vi "test-Vision-Utils-Test2.vi"() -> (3 "All Passed":bool)   [LabVIEW 2019]
uses:
  <vilib>/Rock Robotics/WPI/ThirdParty/JAS_Junk/TrajLib/Rotation_CreateAngle.vi
  <vilib>/Rock Robotics/WPI/ThirdParty/JAS_Junk/TrajLib/Rotation_GetAngleCosSin.vi
  <vilib>/Rock Robotics/WPI/ThirdParty/JAS_Junk/TrajLib/Rotation_UnaryMinus.vi
  <vilib>/Rock Robotics/WPI/ThirdParty/JAS_Junk/TrajLib/Rotation_Minus.vi
  <vilib>/Rock Robotics/WPI/ThirdParty/JAS_Junk/TrajLib/Pose_getRotation.vi
  <vilib>/Rock Robotics/WPI/ThirdParty/JAS_Junk/TrajLib/CompVisionUtil_EstimateFieldToCamera.vi
  <vilib>/Rock Robotics/WPI/ThirdParty/JAS_Junk/TrajLib/Pose_TransformBy.vi
  <vilib>/Rock Robotics/WPI/ThirdParty/JAS_Junk/TrajLib/Rotation_RotateBy.vi
  <vilib>/Rock Robotics/WPI/ThirdParty/JAS_Junk/TrajLib/Transform_Inverse.vi
  <vilib>/Rock Robotics/WPI/ThirdParty/JAS_Junk/TrajLib/Translation_RotateBy.vi
  <vilib>/Rock Robotics/WPI/ThirdParty/JAS_Junk/TrajLib/Translation_Plus.vi
  <vilib>/Rock Robotics/WPI/ThirdParty/JAS_Junk/TrajLib/Rotation_Plus.vi
  <vilib>/Rock Robotics/WPI/ThirdParty/JAS_Junk/TrajLib/Pose_New_TRRO.vi
  <vilib>/Rock Robotics/WPI/ThirdParty/JAS_Junk/TrajLib/Rotation_CreateXY.vi
  <vilib>/Rock Robotics/WPI/ThirdParty/JAS_Junk/TrajLib/Translation_UnaryMinus.vi
  <vilib>/Rock Robotics/WPI/ThirdParty/JAS_Junk/TrajLib/Util_CalcDist.vi
  <vilib>/Rock Robotics/WPI/ThirdParty/JAS_Junk/TrajLib/Trajectory_Library.lvlib
panel:
  out "Test 3":bool
  out "Test 2":bool
  out "Test 1":bool
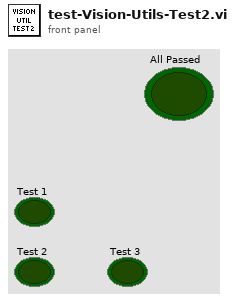
[diagram p1: front panel]
types:
  T1 = typedef "Trajectory_Library.lvlib/ROTATION2D.ctl" = cluster{"VALUE":dbl, "COS":dbl, "SIN":dbl}
  T2 = typedef "Trajectory_Library.lvlib/POSE2D.ctl" = cluster{"TRANSLATION":T3, "ROTATION":T1}
  T3 = typedef "Trajectory_Library.lvlib/TRANSLATION2D.ctl" = cluster{"X":dbl, "Y":dbl}
  T4 = typedef "Trajectory_Library.lvlib/TRANSFORM2D.ctl" = cluster{"TRANSLATION":T3, "ROTATION":T1}
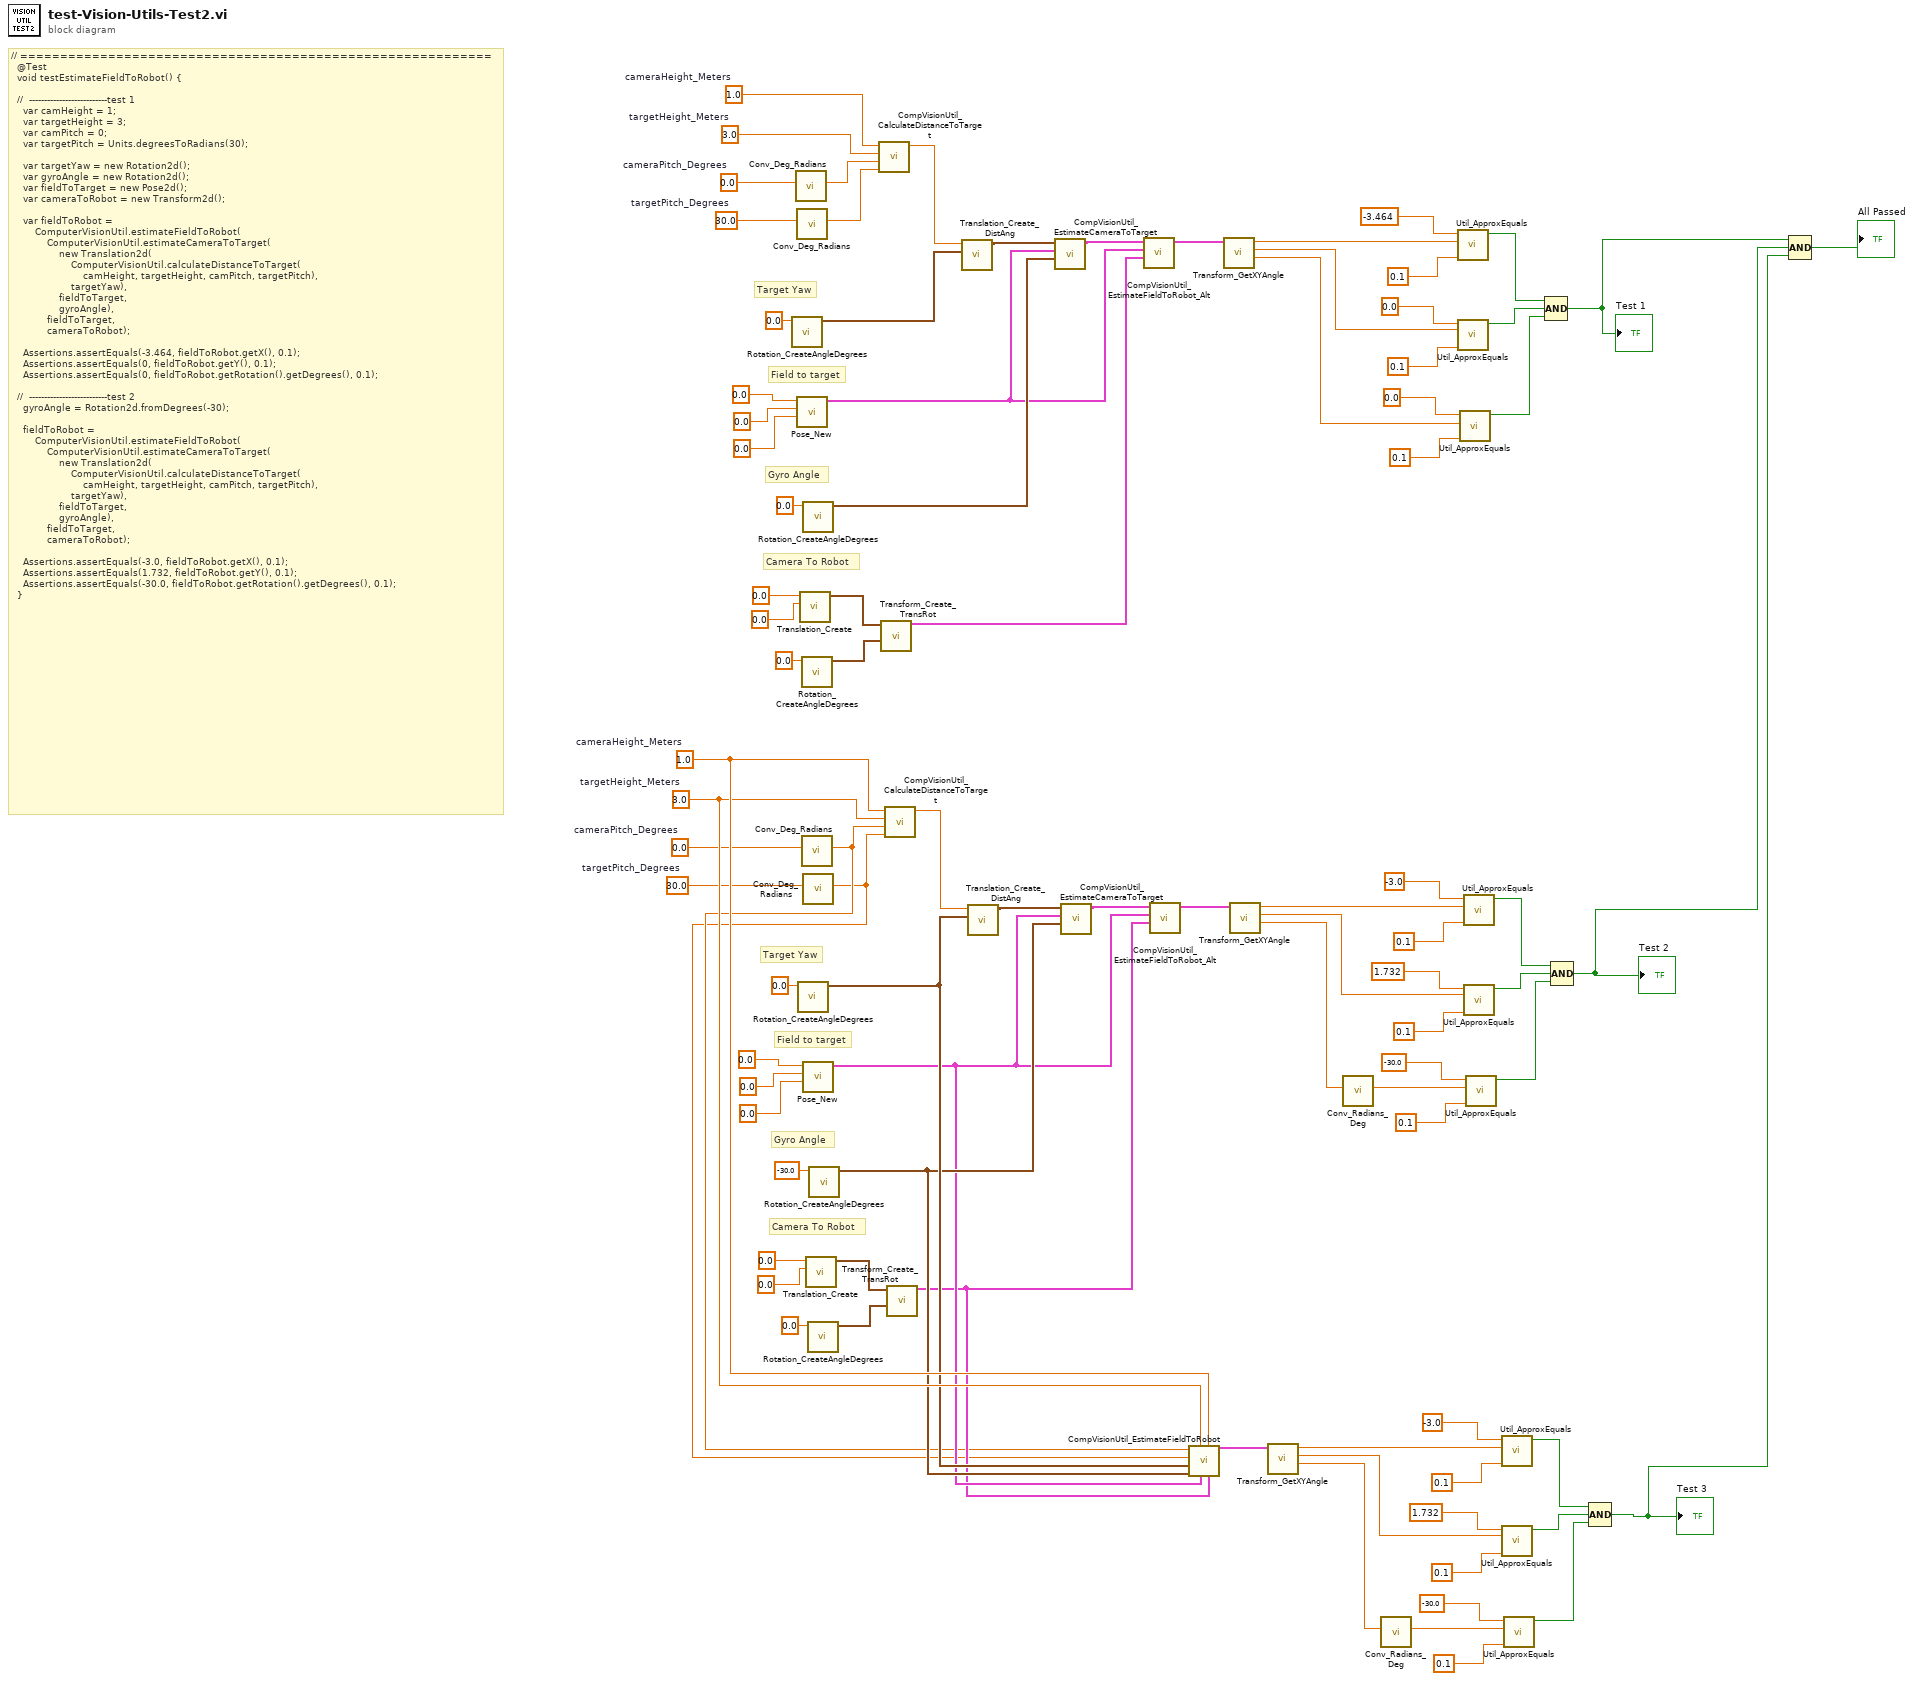
[diagram p0: block diagram]
diagram:
  w11 = 1.0  # cameraHeight_Meters
  w10 = 3.0  # targetHeight_Meters
  w9 = 0.0  # cameraPitch_Degrees
  w8 = 30.0  # targetPitch_Degrees
  w87 = 1.0  # cameraHeight_Meters
  w88 = 3.0  # targetHeight_Meters
  w86 = 0.0  # cameraPitch_Degrees
  w85 = 30.0  # targetPitch_Degrees
  # "Camera To Robot"
  # "Field to target"
  # "Gyro Angle"
  # "Target Yaw"
  # "Camera To Robot"
  # "Field to target"
  # "Gyro Angle"
  # "Target Yaw"
  # "// ===========================================================\n  @Test\n  void testEstimateFieldToRobot() {\n\n  //  --------------------------test 1\n    var camHeight = 1;\n    var targetHeight = 3;\n    var camPitch = 0;\n    var targetPitch = Units.degreesToRadians(30);\n\n    var targetYaw = new Rotation2d();\n    var gyroAngle = new Rotation2d();\n    var fieldToTarget = new Pose2d();\n    var cameraToRobot = new Transform2d();\n\n    var fieldToRobot =\n        ComputerVisionUtil.estimateFieldToRobot(\n            ComputerVisionUtil.estimateCameraToTarget(\n                new Translation2d(\n                    ComputerVisionUtil.calculateDistanceToTarget(\n                        camHeight, targetHeight, camPitch, targetPitch),\n                    targetYaw),\n                fieldToTarget,\n                gyroAngle),\n            fieldToTarget,\n            cameraToRobot);\n\n    Assertions.assertEquals(-3.464, fieldToRobot.getX(), 0.1);\n    Assertions.assertEquals(0, fieldToRobot.getY(), 0.1);\n    Assertions.assertEquals(0, fieldToRobot.getRotation().getDegrees(), 0.1);\n\n  //  --------------------------test 2\n    gyroAngle = Rotation2d.fromDegrees(-30);\n\n    fieldToRobot =\n        ComputerVisionUtil.estimateFieldToRobot(\n            ComputerVisionUtil.estimateCameraToTarget(\n                new Translation2d(\n                    ComputerVisionUtil.calculateDistanceToTarget(\n                        camHeight, targetHeight, camPitch, targetPitch),\n                    targetYaw),\n                fieldToTarget,\n                gyroAngle),\n            fieldToTarget,\n            cameraToRobot);\n\n    Assertions.assertEquals(-3.0, fieldToRobot.getX(), 0.1);\n    Assertions.assertEquals(1.732, fieldToRobot.getY(), 0.1);\n    Assertions.assertEquals(-30.0, fieldToRobot.getRotation().getDegrees(), 0.1);\n  }"
  n1 = call <vilib>:"Rotation_CreateAngleDegrees.vi"("Angle_Degrees"=0.0) -> ("ROTATION"=w80:T1)  [unwired: 10 in]
  n2 = call <vilib>:"Conv_Deg_Radians.vi"("Degress"=w86) -> ("Radians"=w84:dbl)  [unwired: 10 in]
  n3 = call <vilib>:"Conv_Deg_Radians.vi"("Degress"=w85) -> ("Radians"=w83:dbl)  [unwired: 10 in]
  n4 = call <vilib>:"Pose_New.vi"("Heading"=0.0, "Y"=0.0, "X"=0.0) -> ("out POSe"=w72:T2)  [unwired: 8 in]
  n5 = call <vilib>:"Rotation_CreateAngleDegrees.vi"("Angle_Degrees"=0.0) -> ("ROTATION"=w7:T1)  [unwired: 10 in]
  n6 = call <vilib>:"Translation_Create.vi"("Y"=0.0, "X"=0.0) -> ("TRANSLATION"=w68:T3)  [unwired: 9 in]
  n7 = call <vilib>:"Rotation_CreateAngleDegrees.vi"("Angle_Degrees"=0.0) -> ("ROTATION"=w67:T1)  [unwired: 10 in]
  n8 = call <vilib>:"Conv_Deg_Radians.vi"("Degress"=w9) -> ("Radians"=w2:dbl)  [unwired: 10 in]
  n9 = call <vilib>:"Rotation_CreateAngleDegrees.vi"("Angle_Degrees"=0.0) -> ("ROTATION"=w74:T1)  [unwired: 10 in]
  n10 = call <vilib>:"Conv_Deg_Radians.vi"("Degress"=w8) -> ("Radians"=w1:dbl)  [unwired: 10 in]
  n11 = call <vilib>:"Pose_New.vi"("Heading"=0.0, "Y"=0.0, "X"=0.0) -> ("out POSe"=w5:T2)  [unwired: 8 in]
  n12 = call <vilib>:"Translation_Create.vi"("Y"=0.0, "X"=0.0) -> ("TRANSLATION"=w40:T3)  [unwired: 9 in]
  n13 = call <vilib>:"Rotation_CreateAngleDegrees.vi"("Angle_Degrees"=0.0) -> ("ROTATION"=w39:T1)  [unwired: 10 in]
  n14 = call <vilib>:"Rotation_CreateAngleDegrees.vi"("Angle_Degrees"=-30.0) -> ("ROTATION"=w6:T1)  [unwired: 10 in]
  n15 = call <vilib>:"CompVisionUtil_CalculateDistanceToTarget.vi"("targetPitch_Radians"=w83, "cameraPitch_Radians"=w84, "targetHeight_Meters"=w88, "cameraHeight_Meters"=w87) -> ("DistanceToTarget_Meters"=w79:dbl)  [unwired: 7 in]
  n16 = call <vilib>:"Transform_Create_TransRot.vi"("ROTATION"=w67, "TRANSLATION"=w68) -> ("TRANSFORM"=w66:T4)  [unwired: 9 in]
  n17 = call <vilib>:"CompVisionUtil_CalculateDistanceToTarget.vi"("targetPitch_Radians"=w1, "cameraPitch_Radians"=w2, "targetHeight_Meters"=w10, "cameraHeight_Meters"=w11) -> ("DistanceToTarget_Meters"=w49:dbl)  [unwired: 7 in]
  n18 = call <vilib>:"Transform_Create_TransRot.vi"("ROTATION"=w39, "TRANSLATION"=w40) -> ("TRANSFORM"=w4:T4)  [unwired: 9 in]
  n19 = call <vilib>:"Translation_Create_DistAng.vi"("Angle"=w80, "Dist"=w79) -> ("TRANSLATION"=w78:T3)  [unwired: 9 in]
  n20 = call <vilib>:"Translation_Create_DistAng.vi"("Angle"=w7, "Dist"=w49) -> ("TRANSLATION"=w48:T3)  [unwired: 9 in]
  n21 = call <vilib>:"CompVisionUtil_EstimateCameraToTarget.vi"("GyroAngle"=w74, "FieldToTarget"=w72, "CameraToTargetTranslation"=w78) -> ("EstimateCameraToTarget"=w73:T4)  [unwired: 8 in]
  n22 = call <vilib>:"CompVisionUtil_EstimateCameraToTarget.vi"("GyroAngle"=w6, "FieldToTarget"=w5, "CameraToTargetTranslation"=w48) -> ("EstimateCameraToTarget"=w44:T4)  [unwired: 8 in]
  n23 = call <vilib>:"CompVisionUtil_EstimateFieldToRobot_Alt.vi"("CameraToRobot"=w66, "FieldToTarget"=w72, "CameraToTarget"=w73) -> ("EstimatedFieldToRobot"=w65:T4)  [unwired: 8 in]
  n24 = call <vilib>:"CompVisionUtil_EstimateFieldToRobot_Alt.vi"("CameraToRobot"=w4, "FieldToTarget"=w5, "CameraToTarget"=w44) -> ("EstimatedFieldToRobot"=w38:T4)  [unwired: 8 in]
  n25 = call <vilib>:"CompVisionUtil_EstimateFieldToRobot.vi"("CameraToRobot"=w4, "cameraHeight_Meters"=w11, "FieldToTarget"=w5, "targetHeight_Meters"=w10, "GyroAngle"=w6, "TargetYaw"=w7, "targetPitch_Radians"=w1, "cameraPitch_Radians"=w2) -> ("EstimateFieldToRobot"=w12:T2)  [unwired: 3 in]
  n26 = call <vilib>:"Transform_GetXYAngle.vi"("inTRANSFORM"=w65) -> ("Angle"=w55:dbl, "Y"=w56:dbl, "X"=w64:dbl)  [unwired: 8 in]
  n27 = call <vilib>:"Transform_GetXYAngle.vi"("inTRANSFORM"=w38) -> ("Angle"=w27:dbl, "Y"=w29:dbl, "X"=w37:dbl)  [unwired: 8 in]
  n28 = call <vilib>:"Transform_GetXYAngle.vi"("inTRANSFORM"=w12) -> ("Angle"=w13:dbl, "Y"=w15:dbl, "X"=w23:dbl)  [unwired: 8 in]
  n29 = call <vilib>:"Conv_Radians_Deg.vi"("Radians"=w27) -> ("Degrees"=w28:dbl)  [unwired: 10 in]
  n30 = call <vilib>:"Conv_Radians_Deg.vi"("Radians"=w13) -> ("Degrees"=w14:dbl)  [unwired: 10 in]
  n31 = call <vilib>:"Util_ApproxEquals.vi"("Tolerance"=0.1, "Value 2"=w64, "Value 1"=-3.464 ("y")) -> ("ApproxEquals"=w59:bool)  [unwired: 8 in]
  n32 = call <vilib>:"Util_ApproxEquals.vi"("Tolerance"=0.1, "Value 2"=w56, "Value 1"=0.0 ("y")) -> ("ApproxEquals"=w58:bool)  [unwired: 8 in]
  n33 = call <vilib>:"Util_ApproxEquals.vi"("Tolerance"=0.1, "Value 2"=w55, "Value 1"=0.0 ("y")) -> ("ApproxEquals"=w57:bool)  [unwired: 8 in]
  n34 = call <vilib>:"Util_ApproxEquals.vi"("Tolerance"=0.1, "Value 2"=w37, "Value 1"=-3.0 ("y")) -> ("ApproxEquals"=w32:bool)  [unwired: 8 in]
  n35 = call <vilib>:"Util_ApproxEquals.vi"("Tolerance"=0.1, "Value 2"=w29, "Value 1"=1.732 ("y")) -> ("ApproxEquals"=w31:bool)  [unwired: 8 in]
  n36 = call <vilib>:"Util_ApproxEquals.vi"("Tolerance"=0.1, "Value 2"=w28, "Value 1"=-30.0 ("y")) -> ("ApproxEquals"=w30:bool)  [unwired: 8 in]
  n37 = call <vilib>:"Util_ApproxEquals.vi"("Tolerance"=0.1, "Value 2"=w23, "Value 1"=-3.0 ("y")) -> ("ApproxEquals"=w18:bool)  [unwired: 8 in]
  n38 = call <vilib>:"Util_ApproxEquals.vi"("Tolerance"=0.1, "Value 2"=w15, "Value 1"=1.732 ("y")) -> ("ApproxEquals"=w17:bool)  [unwired: 8 in]
  n39 = call <vilib>:"Util_ApproxEquals.vi"("Tolerance"=0.1, "Value 2"=w14, "Value 1"=-30.0 ("y")) -> ("ApproxEquals"=w16:bool)  [unwired: 8 in]
  n40 = Compound Arithmetic op=AND(w59, w58, w57) -> (w54:bool)
  "Test 1" <- w54
  n41 = Compound Arithmetic op=AND(w32, w31, w30) -> (w26:bool)
  "Test 2" <- w26
  n42 = Compound Arithmetic op=AND(w18, w17, w16) -> (w3:bool)
  "Test 3" <- w3
  n43 = Compound Arithmetic op=AND(w54, w26, w3) -> (→"All Passed":bool)
